vi "Set Title Icon.vi"(8 "Error In":errorcluster, 10 "Icon Path":path, 11 "VI Reference":refnum<vi>) -> (0 "Error Out":errorcluster)   [LabVIEW 2021, in "Seq Edit Quick Drop.lvlib"]
uses:
  Seq Edit Quick Drop.lvlib
  user32.dll
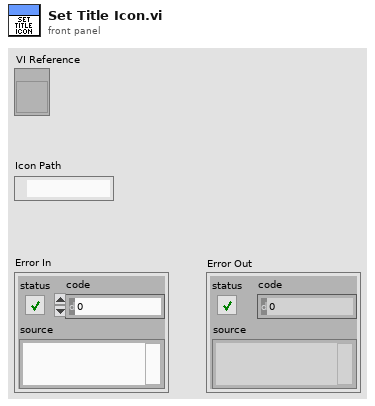
[diagram p1: front panel]
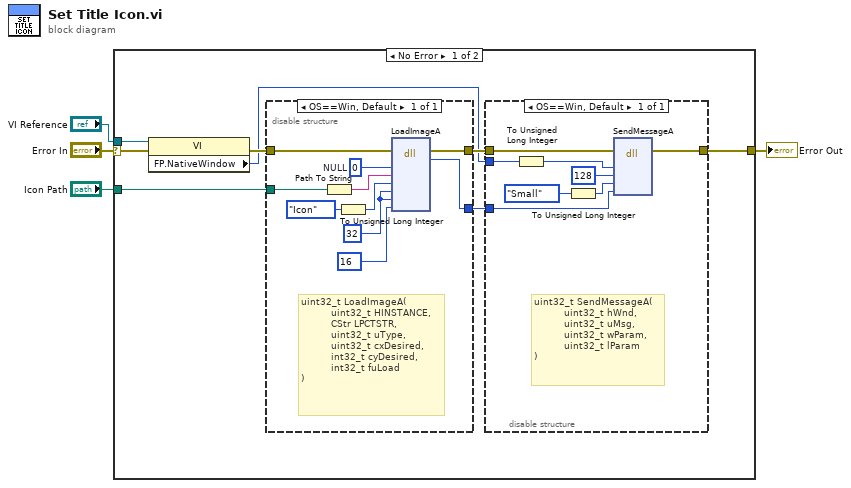
[diagram p0: block diagram]
diagram:
  n1 = case shown="No Error" "Error In" {
    selector: "Error In" -> [w5 w31]
    tunnel: "Icon Path" -> [w11 _]
    tunnel: "VI Reference" -> [w10 _]
    tunnel: [w9 w31] -> w1
    frame No Error {
      n2 = property class="VI"(reference=w10, error in=w5) -> (error out=w8:errorcluster, "FP.NativeWindow"=w7:u64)  [unwired: 1 out]
      n3 = disable-structure shown="OS==Win, Default" {
        disable-tunnel: w11 -> [w27]
        disable-tunnel: w8 -> [w25]
        disable-tunnel: [w23] -> w6
        disable-tunnel: [w22] -> w12
        frame condition #0 (active) {
          w29 = u32 32 ("cxDesired")
          w30 = u32 0  # NULL
          # "uint32_t LoadImageA(\n          uint32_t HINSTANCE,\n          CStr LPCTSTR,\n          uint32_t uType,\n          uint32_t cxDesired,\n          int32_t cyDesired,\n          int32_t fuLoad\n)"
          n4 = Path To String(path=w27) -> (string=w26:string)
          n5 = To Unsigned Long Integer(number=enum16{"Bitmap", "Icon", "Cursor"}."Icon") -> (unsigned 32bit integer=w21:u32)
          n6 = dll-call lib="user32.dll" fn="LoadImageA" label="LoadImage"(error in=w25, "HINSTANCE"=w30, "LPCTSTR"=w26, "uType"=w21, "cxDesired"=w29, "cyDesired"=w29, "fuLoad"=16) -> (error out=w22:errorcluster, "ImageHandle"=w23:u32)  [unwired: 8 in, 1 out]
        }
      }
      n7 = disable-structure shown="OS==Win, Default" {
        disable-tunnel: [w20] -> w9
        disable-tunnel: w7 -> [w18]
        disable-tunnel: w6 -> [w16]
        disable-tunnel: w12 -> [w15]
        frame condition #0 (active) {
          # "uint32_t SendMessageA(\n          uint32_t hWnd,\n          uint32_t uMsg,\n          uint32_t wParam,\n          uint32_t lParam\n)"
          n8 = To Unsigned Long Integer(number=w18) -> (unsigned 32bit integer=w13:u32)
          n9 = To Unsigned Long Integer(number=enum32{"Small", "Big"}."Small") -> (unsigned 32bit integer=w14:u32)
          n10 = dll-call lib="user32.dll" fn="SendMessageA" label="SendMessage"(error in=w15, "hWnd"=w13, "uMsg"=u32 128 ("dimension size"), "wParam"=w14, "lParam"=w16) -> (error out=w20:errorcluster)  [unwired: 7 in, 1 out]
        }
      }
    }
    frame Error {
    }
  }
  "Error Out" <- w1
